vi "from string.vi"(8 "error in":errorcluster, 9 "data":string, 10 "version":string, 11 "Channel configuration":refnum<class "Channel configuration.lvclass">) -> (0 "error out":errorcluster, 3 "Channel configuration out":refnum<class "Channel configuration.lvclass">)   [LabVIEW 2025, in "Abstract Engine.lvlib" / "Channel configuration.lvclass"]
doc: "Provides an interface for loading a module configuration from a file or other serialized data source. It is recommended that all children of this class store data in two sets--data required for its own initialization, and any data required for parent initialization--and that each implementation uses the <b>Call Parent Method</b> primitive to de-serialize parent information.Copyright 2017 National Instruments Corporation\n\nLicensed under the Apache License, Version 2.0 (the \"License\"); you may not use this file except in compliance with the License. You may obtain a copy of the License at http://www.apache.org/licenses/LICENSE-2.0\nUnless required by applicable law or agreed to in writing, software distributed under the License is distributed on an \"AS IS\" BASIS, WITHOUT WARRANTIES OR CONDITIONS OF ANY KIND, either express or implied. See the License for the specific language governing permissions and limitations under the License."
uses:
  Channel configuration.lvclass
  Default Channel.ctl
  Channel configuration.lvclass/Channel configuration.ctl
  Users/Public/Documents/Sandia National Labs/TSS Plugin/CEF.lvlibp/serializable configuration/CEF_serializable configuration.lvclass
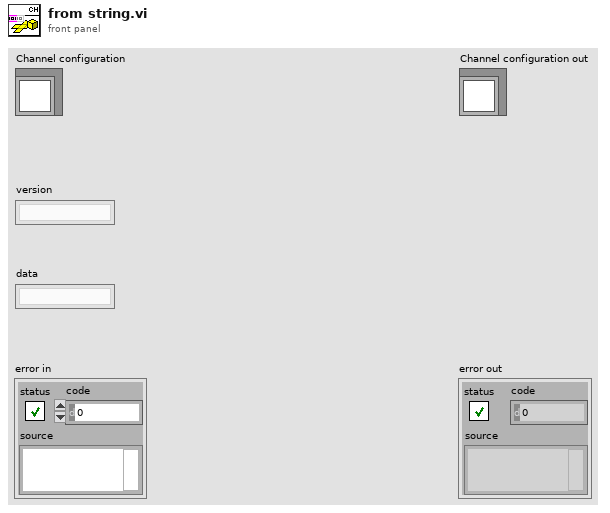
[diagram p1: front panel]
types:
  T1 = typedef "Abstract Engine.lvlib/Channel configuration.lvclass/Default Channel.ctl" = cluster{"Address":string, "SW Alias":string, "Description":string, "Enabled":bool, "Type":string}
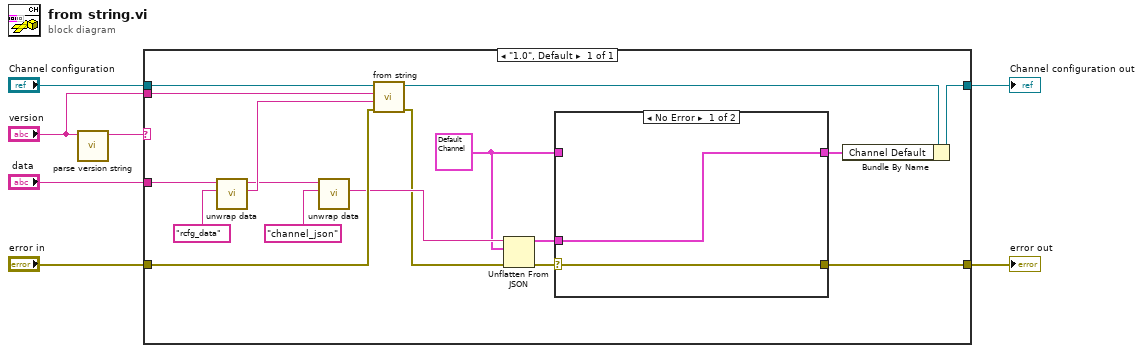
[diagram p0: block diagram]
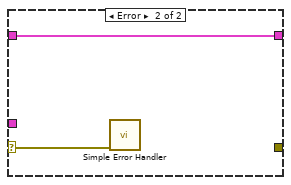
[diagram p2: hidden frame]
diagram:
  n1 = call "parse version string.vi"("full version"="version") -> ("major.minor version"=w3:string)  [unwired: 7 in, 3 out]
  n2 = case shown="\"1.0\", Default" w3 {
    tunnel: "Channel configuration" -> [w24]
    tunnel: [w16] -> w6
    tunnel: "data" -> [w22]
    tunnel: "error in" -> [w17]
    tunnel: "version" -> [w13]
    tunnel: [w8] -> w1
    frame "1.0", Default {
      w10 = T1 {"Address"="None", "SW Alias"="", "Description"="", "Enabled"=TRUE, "Type"="Type = Class \n"} ("Default Engine")
      n3 = call "unwrap data.vi"("identifier"="rcfg_data" ("additional identifier"), "data to unwrap"=w22) -> ("unwrapped data"=w20:string, "remaining string"=w19:string)  [unwired: 8 in]
      n4 = call "unwrap data.vi"("identifier"="channel_json" ("additional identifier"), "data to unwrap"=w19) -> ("unwrapped data"=w15:string)  [unwired: 8 in, 1 out]
      n5 = call-parent "from string.vi"("error in"=w17, "data"=w20, "version"=w13, "CEF_Configuration in"=w24) -> ("error out"=w14:errorcluster, "CEF_Configuration out"=w23:refnum<class "Channel configuration.lvclass">)  [unwired: 6 in]
      n6 = Unflatten From JSON(JSON string=w15, type and defaults=w10, error in (no error)=w14) -> (value=w11:T1, error out=w12:errorcluster)  [unwired: 4 in]
      n7 = case shown="No Error" w12 {
        selector: w12 -> [w25 w27]
        tunnel: w11 -> [w26 _]
        tunnel: [w26 w28] -> w9
        tunnel: w10 -> [_ w28]
        tunnel: [w25 _] -> w8
        frame No Error {
        }
        frame Error {
          n8 = call <vilib>:"Simple Error Handler.vi"("error in (no error)"=w27) -> ()  [unwired: 4 in, 5 out]
        }
      }
      n9 = Bundle By Name(cluster=w23, "Channel Default"=w9) -> (w16:refnum<class "Channel configuration.lvclass">)
    }
  }
  "error out" <- w1
  "Channel configuration out" <- w6
